vi "Main.vi"() -> ()   [LabVIEW 2021]
doc: "This Continuous Measurement sample project is based on the Queued Message Handler template.\n\nThe Event Handling Loop generates messages based on user interface actions.\n\nThe Message Handling Loop processes messages generated by the Event Handling Loop, or by other messages. There are also Acquisition and Logging message handling loop subVIs, and a chart updating loop."
uses:
  controls/Acquisition Status.ctl
  controls/UI Data.ctl
  controls/Acquired Data.ctl
  controls/UI State.ctl
  support/Message Queue/Enqueue Message (Single).vi
  support/Message Queue/Enqueue Message (Array).vi
  <vilib>/Utility/error.llb/Error Cluster From Error Code.vi
  <vilib>/ErrorRing/Error Ring.xnode
  Acquisition/Acquisition.lvlib
  Logging/Logging.lvlib
  Settings/Settings.lvlib
  support/User Event - Stop/User Event - Stop.lvlib
  support/Message Queue/Message Queue.lvlib
  Settings/Settings Dialog.vi
  Diagnostics/Diagnostics.lvlib
panel:
  out "Data":waveform(dbl)[](graph)
  in  "Save Now":bool
  in  "Settings":bool
  in  "Start":bool
  in  "Stop":bool
  out "Acquisition status":T1
  out "Status":string
  in  "Exit":bool
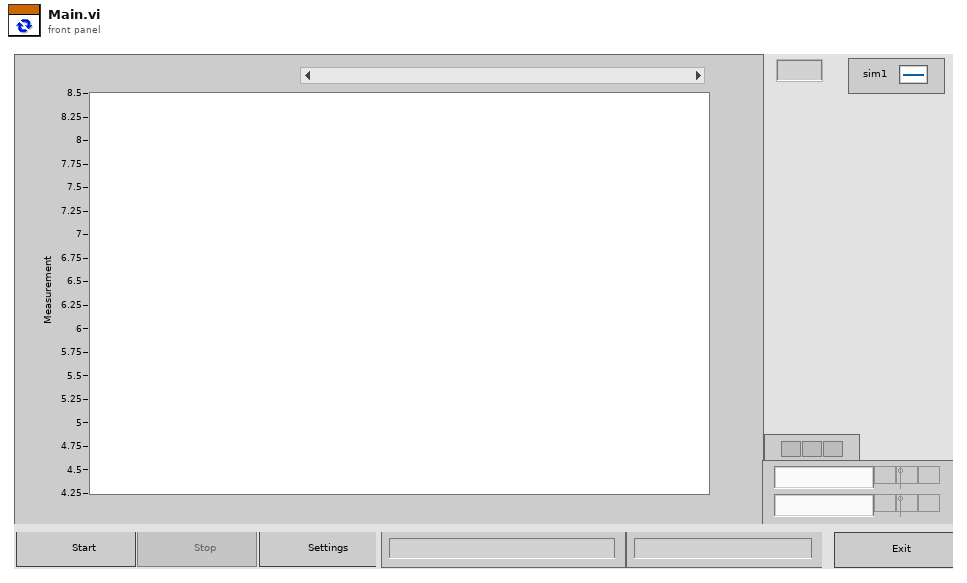
[diagram p1: front panel]
types:
  T1 = typedef "Acquisition Status.ctl" = string
  T2 = typedef "UI State.ctl" = enum16{"Idle", "Acquiring and Logging", "Waiting for Exit", "Waiting for Exit (Acq Stopped)", "Waiting for Exit (Log Stopped)", "Waiting for Stop", "Waiting for Stop (Acq Stopped)", "Waiting for Stop (Log Stopped)"}
  T3 = typedef "Acquired Data.ctl" = cluster{"Waveform Array":waveform(dbl)[]}
  T4 = typedef "UI Data.ctl" = cluster{"Start Ref":refnum<vi>, "Stop Ref":refnum<vi>, "Settings Ref":refnum<vi>, "Exit Ref":refnum<vi>, "Status Ref":refnum<vi>, "Data Ref":refnum<vi>, "Save Ref":refnum<vi>}
  T5 = typedef "Message Queue.lvlib/All Message Queues.ctl" = cluster{"UI":refnum<queue>, "Acquisition":refnum<queue>, "Logging":refnum<queue>, "Diagnostic":refnum<queue>}
  T6 = typedef "Settings.lvlib/Settings.ctl" = cluster{"IO":T7, "Log":T13, "Debug":T14}
  T7 = typedef "Acquisition.lvlib/Hardware Configuration.ctl" = cluster{"Channel Settings":T8[], "Sensor Intervals":T10[], "Sensor Token":T12}
  T8 = typedef "Acquisition.lvlib/Channel Settings.ctl" = cluster{"Name":string, "Terminal Information":cluster{"IO Device":T9, "Channel Number":i32}, "Calibration Information":cluster{"Excitation Voltage":dbl, "Calibration Factor":dbl, "Zero Value":dbl, "Calibration Formula":string}}
  T9 = typedef "Acquisition.lvlib/IO Device.ctl" = enum16{"none", "9219", "9401"}
  T10 = typedef "Interval Timer.lvlib/Repeat Interval.ctl" = cluster{"Interval":T11, "Count":i32}
  T11 = typedef "Interval Timer.lvlib/Interval Length.ctl" = enum16{"Manual control", "1 second", "10 seconds", "30 seconds", "60 seconds", "600 seconds", "1200 seconds", "3600 seconds"}
  T12 = typedef "Interval Timer.lvlib/Interval Token.ctl" = cluster{"Next reading in ms":u32, "Interval Index":i32, "Interval Occurrence":i32}
  T13 = typedef "Logging.lvlib/Logging Configuration.ctl" = cluster{"Path":path, "Spreadsheet":refnum<file>, "Append":bool}
  T14 = typedef "Diagnostics.lvlib/Diagnostics Configuration.ctl" = cluster{"Messages":refnum<file>}
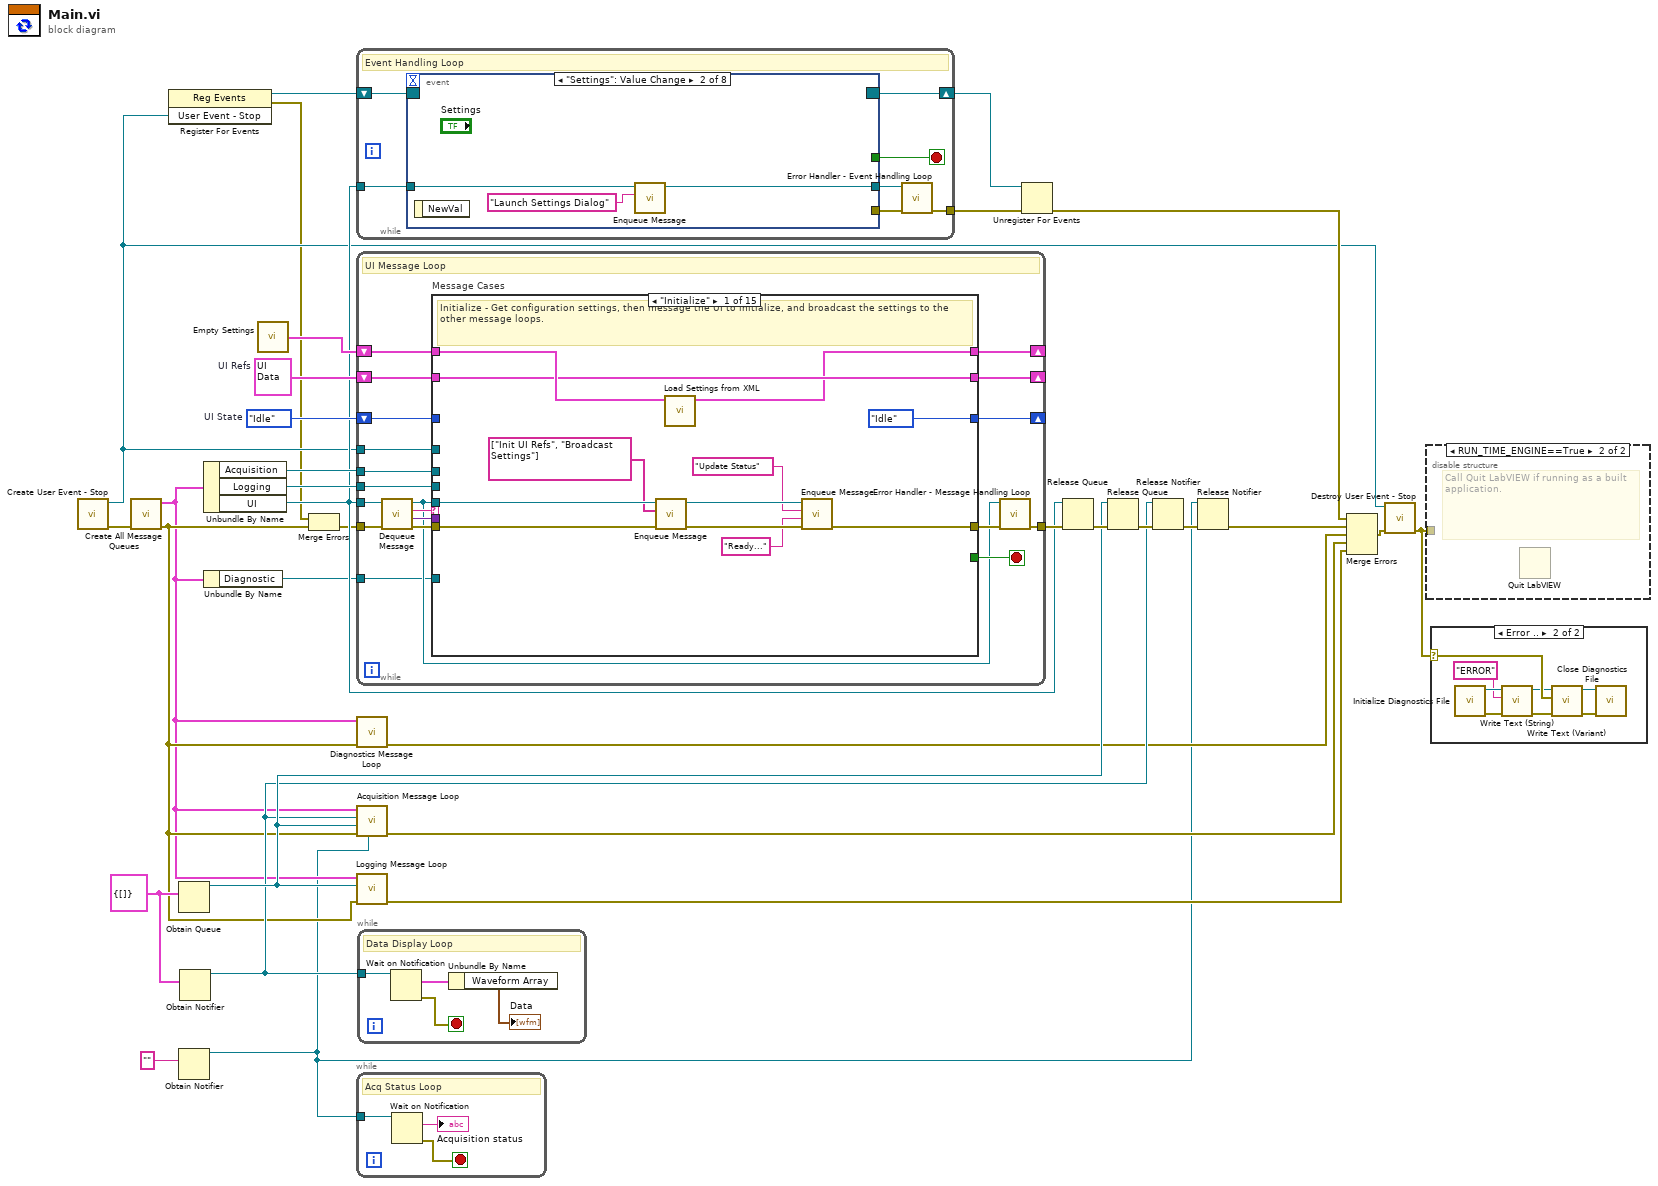
[diagram p0: block diagram]
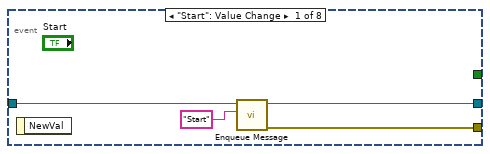
[diagram p4: hidden frame]
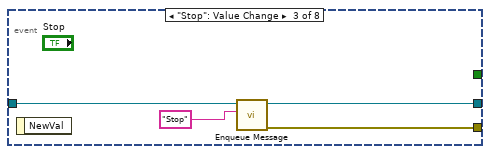
[diagram p5: hidden frame]
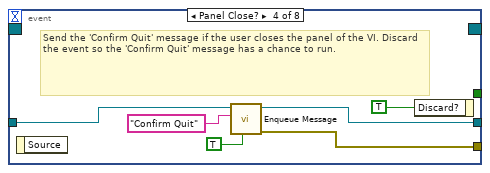
[diagram p6: hidden frame]
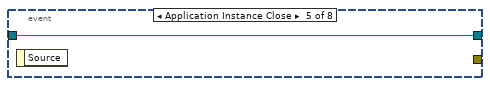
[diagram p7: hidden frame]
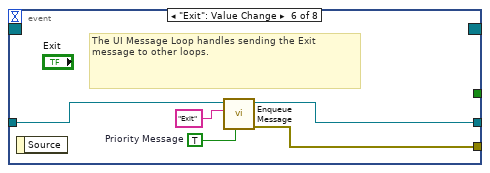
[diagram p8: hidden frame]
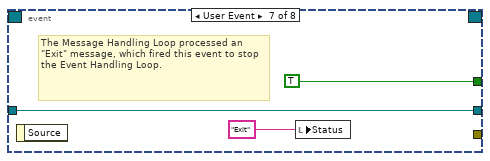
[diagram p9: hidden frame]
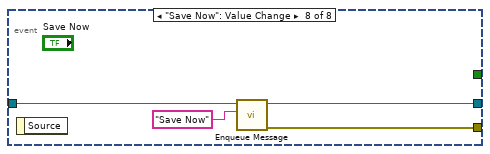
[diagram p10: hidden frame]
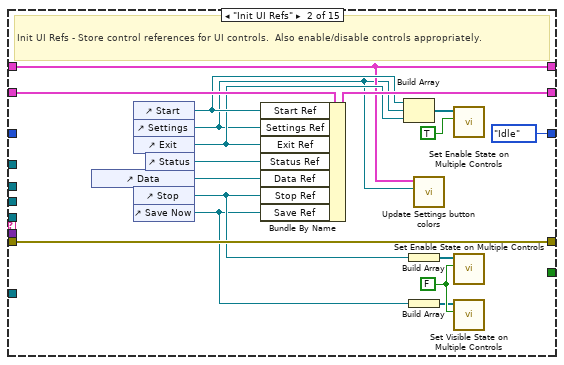
[diagram p11: hidden frame]
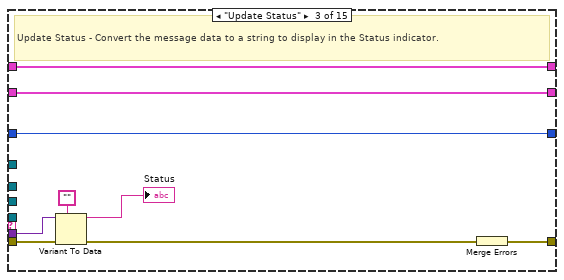
[diagram p12: hidden frame]
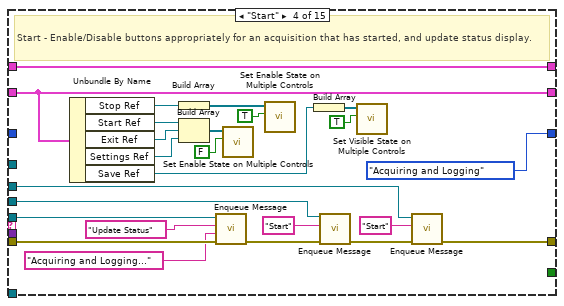
[diagram p13: hidden frame]
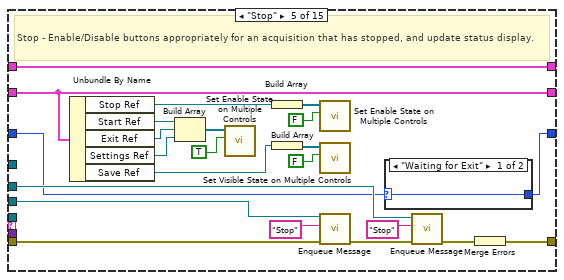
[diagram p14: hidden frame]
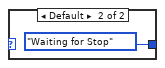
[diagram p15: hidden frame]
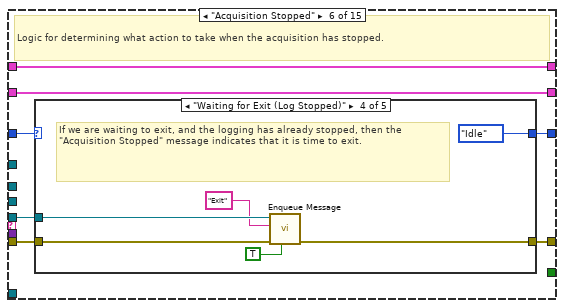
[diagram p16: hidden frame]
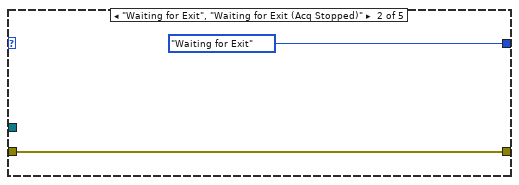
[diagram p18: hidden frame]
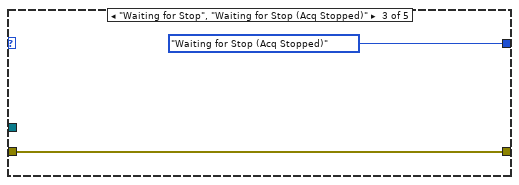
[diagram p19: hidden frame]
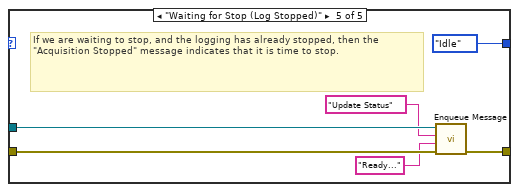
[diagram p20: hidden frame]
diagram:
  w21 = UI_State."Idle"  # UI State
  w14 = T3 {"Waveform Array"=[]}
  w24 = T4 {"Start Ref"=refnum, "Stop Ref"=refnum, "Settings Ref"=refnum, "Exit Ref"=refnum, "Status Ref"=refnum, "Data Ref"=refnum, "Save Ref"=refnum}  # UI Refs
  n1 = call "Create User Event - Stop.vi"() -> ("error out"=w29:errorcluster, "User Event - Stop"=w12:refnum<user-event>)  [unwired: 10 in]
  n2 = call "Create All Message Queues.vi"("error in (no error)"=w29) -> ("error out"=w8:errorcluster, "Message Queues out"=w7:T5)  [unwired: 9 in]
  n3 = register-events(w12) -> (reference out=w13:refnum<event-registration>, error out=w10:errorcluster)  [unwired: 2 in]
  n4 = Obtain Queue(element data type=w14) -> (queue out=w16:refnum<queue>)  [unwired: 4 in, 2 out]
  n5 = Obtain Notifier(notification data type=T1 "") -> (notifier out=w1:refnum<notifier>)  [unwired: 3 in, 2 out]
  n6 = Obtain Notifier(notification data type=w14) -> (notifier out=w15:refnum<notifier>)  [unwired: 3 in, 2 out]
  n7 = Unbundle By Name(w7) -> ("Acquisition"=w23:refnum<queue>, "Logging"=w22:refnum<queue>, "UI"=w19:refnum<queue>)
  n8 = Unbundle By Name(w7) -> ("Diagnostic"=w9:refnum<queue>)
  n9 = call "Empty Settings.vi"() -> ("Settings"=w27:T6)
  n10 = Merge Errors(w10, w8) -> (w11:errorcluster)
  n11 = while {
    tunnel: w19 -> [w38]
    tunnel: [w35] -> w31
    shift-right: [w37] -> w25
    shift-left: w13 -> [w39]
    stop <- w36 stop-if-true
    # "Event Handling Loop"
    n12 = event shown="[1] \"Settings\": Value Change" {
      selector: w39 -> [_ _ _ _ _ _ _ _]
      dyn-events: [_ _ _ _ _ _ _ _] -> w37
      timeout: _ -> [_ _ _ _ _ _ _ _]
      tunnel: [_ _ _ _ _ _ TRUE ("Discard?") _] -> w36
      tunnel: w38 -> [w43 w45 w49 w54 w57 w59 w63 w69]
      tunnel: [w41 _ w48 w52 _ w62 _ w67] -> w34
      tunnel: [w40 w44 w47 w53 w57 w58 w63 w68] -> w33
      event "Start": Value Change {
        n13 = event-data() -> ()  [unwired: 1 in, 1 out]
        n14 = call-poly "Enqueue Message.vi"("Message"="Start", "Message Queue"=w43) -> ("error out"=w41:errorcluster, "dup Message Queue"=w40:refnum<queue>)  [unwired: 8 in]
      }
      event "Settings": Value Change {
        n15 = event-data() -> ()  [unwired: 1 in, 1 out]
        n16 = call-poly "Enqueue Message.vi"("Message"="Launch Settings Dialog", "Message Queue"=w45) -> ("dup Message Queue"=w44:refnum<queue>)  [unwired: 8 in, 1 out]
      }
      event "Stop": Value Change {
        n17 = event-data() -> ()  [unwired: 1 in, 1 out]
        n18 = call-poly "Enqueue Message.vi"("Message"="Stop", "Message Queue"=w49) -> ("error out"=w48:errorcluster, "dup Message Queue"=w47:refnum<queue>)  [unwired: 8 in]
      }
      event Panel Close? {
        # "Send the 'Confirm Quit' message if the user closes the panel of the VI. Discard the event so the 'Confirm Quit' message has a chance to run."
        n19 = event-data() -> ()  [unwired: 1 in, 1 out]
        n20 = call-poly "Enqueue Message.vi"("Priority Message? (F)"=TRUE, "Message"="Confirm Quit", "Message Queue"=w54) -> ("error out"=w52:errorcluster, "dup Message Queue"=w53:refnum<queue>)  [unwired: 7 in]
        n21 = event-data("Discard?"=TRUE) -> ()  [unwired: 1 in, 1 out]
      }
      event Application Instance Close {
        n22 = event-data() -> ()  [unwired: 1 in, 1 out]
      }
      event "Exit": Value Change {
        w60 = TRUE  # Priority Message
        # "The UI Message Loop handles sending the Exit message to other loops."
        n23 = event-data() -> ()  [unwired: 1 in, 1 out]
        n24 = call-poly "Enqueue Message.vi"("Priority Message? (F)"=w60, "Message"="Exit", "Message Queue"=w59) -> ("error out"=w62:errorcluster, "dup Message Queue"=w58:refnum<queue>)  [unwired: 7 in]
      }
      event User Event {
        # "The Message Handling Loop processed an \"Exit\" message, which fired this event to stop the Event Handling Loop."
        n25 = event-data() -> ()  [unwired: 1 in, 1 out]
        n26 = local write "Status"("Exit" ("Exit String")) -> ()
      }
      event "Save Now": Value Change {
        n27 = event-data() -> ()  [unwired: 1 in, 1 out]
        n28 = call-poly "Enqueue Message.vi"("Message"="Save Now", "Message Queue"=w69) -> ("error out"=w67:errorcluster, "dup Message Queue"=w68:refnum<queue>)  [unwired: 8 in]
      }
    }
    n29 = call "Error Handler - Event Handling Loop.vi"("error in (no error)"=w34, "Message Queue"=w33) -> ("dup error in"=w35:errorcluster)  [unwired: 8 in, 1 out]
  }
  n30 = while {
    tunnel: w19 -> [w82]
    tunnel: w12 -> [w87]
    shift-right: [w81] -> _
    shift-left: w27 -> [w80]
    shift-right: [w78] -> _
    shift-left: w24 -> [w79]
    tunnel: w23 -> [w77]
    tunnel: w22 -> [w76]
    shift-right: [w71] -> _
    shift-left: w21 -> [w72]
    tunnel: w11 -> [w86]
    tunnel: [w75] -> w32
    tunnel: w9 -> [w70]
    stop <- w88 stop-if-true
    # "UI Message Loop"
    n31 = call "Dequeue Message.vi"("error in (no error)"=w86, "Message Queue"=w82) -> ("error out"=w85:errorcluster, "Message Data"=w83:variant, "Message"=w84:string, "dup Message Queue"=w73:refnum<queue>)  [unwired: 6 in]
    n32 = case "Message Cases" shown="\"Initialize\"" w84 {
      selector: w84 -> [_ _ _ _ _ _ _ _ _ _ _ _ _ _ w330]
      tunnel: w73 -> [w93 _ _ w151 _ w179 w204 _ w248 _ w269 _ _ _ _]
      tunnel: w85 -> [w92 w117 w125 w150 w173 w180 w205 w239 w250 w257 w268 w307 w320 w323 _]
      tunnel: [w97 w117 w126 w133 w174 w177 w202 w231 w243 w260 w267 w314 w319 w328 w329] -> w74
      tunnel: [_ _ _ _ _ _ _ _ _ _ _ TRUE _ _ _] -> w88
      tunnel: w83 -> [_ _ w124 _ _ _ _ _ _ w261 _ w305 _ _ _]
      tunnel: w87 -> [_ _ _ _ _ _ _ _ _ _ _ w296 _ _ _]
      tunnel: [w89 w102 w120 w149 w172 w183 w208 w227 w247 w265 w272 w300 w318 w327 w333] -> w81
      tunnel: w80 -> [w100 w102 w120 w149 w172 w183 w208 w227 w251 w265 w272 w300 w318 w327 w333]
      tunnel: w79 -> [w94 w116 w119 w146 w171 w182 w207 w230 w245 w264 w271 w295 w317 w326 w332]
      tunnel: [w94 w113 w119 w146 w171 w182 w207 w230 w245 w264 w271 w295 w317 w326 w332] -> w78
      tunnel: w77 -> [_ _ _ w132 w158 _ _ w238 _ _ _ w313 _ w321 _]
      tunnel: w76 -> [_ _ _ w135 w161 _ _ w237 _ _ _ w312 _ _ _]
      tunnel: w72 -> [_ _ w118 _ w155 w181 w206 w236 w244 w259 w270 _ w316 w325 w331]
      tunnel: [UI_State."Idle" ("UI State") UI_State."Idle" ("UI State") w118 UI_State."Acquiring and Logging" ("UI State") w156 w178 w203 w236 w244 w259 w266 UI_State."Idle" ("UI State") w316 w325 w331] -> w71
      tunnel: w70 -> [_ _ _ _ _ _ _ w235 _ _ _ w303 _ _ _]
      frame "Initialize" {
        # "Initialize - Get configuration settings, then message the UI to initialize, and broadcast the settings to the other message loops."
        n33 = call-poly "Enqueue Message.vi"("error in (no error)"=w92, "Message Array"=string[] ["Init UI Refs", "Broadcast Settings"], "Message Queue"=w93) -> ("error out"=w99:errorcluster, "dup Message Queue"=w98:refnum<queue>)  [unwired: 7 in]
        n34 = call "Load Settings from XML.vi"("Settings in"=w100) -> ("Settings out"=w89:T6)  [unwired: 9 in, 1 out]
        n35 = call-poly "Enqueue Message.vi"("error in (no error)"=w99, "Message Data"="Ready..." ("Ready..."), "Message"="Update Status", "Message Queue"=w98) -> ("error out"=w97:errorcluster)  [unwired: 6 in, 1 out]
      }
      frame "Init UI Refs" {
        w105 = FALSE ("Enable?")
        # "Init UI Refs - Store control references for UI controls.  Also enable/disable controls appropriately."
        n36 = control-ref of="Data"() -> (w114:refnum<vi>)
        n37 = control-ref of="Start"() -> (w109:refnum<vi>)
        n38 = control-ref of="Settings"() -> (w101:refnum<vi>)
        n39 = control-ref of="Exit"() -> (w108:refnum<vi>)
        n40 = control-ref of="Stop"() -> (w106:refnum<vi>)
        n41 = control-ref of="Save Now"() -> (w103:refnum<vi>)
        n42 = control-ref of="Status"() -> (w115:refnum<vi>)
        n43 = Bundle By Name(cluster=w116, "Start Ref"=w109, "Settings Ref"=w101, "Exit Ref"=w108, "Status Ref"=w115, "Data Ref"=w114, "Stop Ref"=w106, "Save Ref"=w103) -> (w113:T4)
        n44 = Build Array(w109, w101, w108) -> (w111:refnum<vi>[])
        n45 = Build Array(w106) -> (w110:refnum<vi>[])
        n46 = Build Array(w103) -> (w104:refnum<vi>[])
        n47 = call "Update Settings button colors.vi"("Bool Refnum"=w101, "Settings in"=w102) -> ()  [unwired: 8 in, 2 out]
        n48 = call "Set Enable State on Multiple Controls.vi"("Enable?"=TRUE, "Controls"=w111) -> ()  [unwired: 9 in, 1 out]
        n49 = call "Set Enable State on Multiple Controls.vi"("Enable?"=w105, "Controls"=w110) -> ()  [unwired: 9 in, 1 out]
        n50 = call "Set Visible State on Multiple Controls.vi"("Visible?"=w105, "Controls"=w104) -> ()  [unwired: 10 in]
      }
      frame "Update Status" {
        # "Update Status - Convert the message data to a string to display in the Status indicator."
        n51 = Variant To Data(error in=w125, type="", Variant=w124) -> (data=→"Status":string, error out=w122:errorcluster)
        n52 = Merge Errors(w122) -> (w126:errorcluster)
      }
      frame "Start" {
        # "Start - Enable/Disable buttons appropriately for an acquisition that has started, and update status display."
        n53 = Unbundle By Name(w146) -> ("Stop Ref"=w141:refnum<vi>, "Start Ref"=w140:refnum<vi>, "Exit Ref"=w139:refnum<vi>, "Settings Ref"=w138:refnum<vi>, "Save Ref"=w128:refnum<vi>)
        n54 = Build Array(w141) -> (w143:refnum<vi>[])
        n55 = Build Array(w140, w139, w138) -> (w144:refnum<vi>[])
        n56 = call-poly "Enqueue Message.vi"("error in (no error)"=w150, "Message Data"="Acquiring and Logging..." ("Acquiring and Logging..."), "Message"="Update Status", "Message Queue"=w151) -> ("error out"=w137:errorcluster)  [unwired: 6 in, 1 out]
        n57 = call "Set Enable State on Multiple Controls.vi"("Enable?"=FALSE, "Controls"=w144) -> ()  [unwired: 9 in, 1 out]
        n58 = call "Set Enable State on Multiple Controls.vi"("Enable?"=TRUE, "Controls"=w143) -> ()  [unwired: 9 in, 1 out]
        n59 = Build Array(w128) -> (w129:refnum<vi>[])
        n60 = call-poly "Enqueue Message.vi"("error in (no error)"=w137, "Message"="Start", "Message Queue"=w135) -> ("error out"=w134:errorcluster)  [unwired: 7 in, 1 out]
        n61 = call "Set Visible State on Multiple Controls.vi"("Visible?"=TRUE ("Visble?"), "Controls"=w129) -> ()  [unwired: 10 in]
        n62 = call-poly "Enqueue Message.vi"("error in (no error)"=w134, "Message"="Start", "Message Queue"=w132) -> ("error out"=w133:errorcluster)  [unwired: 7 in, 1 out]
      }
      frame "Stop" {
        # "Stop - Enable/Disable buttons appropriately for an acquisition that has stopped, and update status display."
        n63 = Unbundle By Name(w171) -> ("Stop Ref"=w166:refnum<vi>, "Start Ref"=w165:refnum<vi>, "Exit Ref"=w164:refnum<vi>, "Settings Ref"=w163:refnum<vi>, "Save Ref"=w152:refnum<vi>)
        n64 = Build Array(w165, w164, w163) -> (w169:refnum<vi>[])
        n65 = call "Set Enable State on Multiple Controls.vi"("Enable?"=TRUE, "Controls"=w169) -> ()  [unwired: 9 in, 1 out]
        n66 = Build Array(w166) -> (w168:refnum<vi>[])
        n67 = Build Array(w152) -> (w154:refnum<vi>[])
        n68 = call "Set Enable State on Multiple Controls.vi"("Enable?"=FALSE, "Controls"=w168) -> ()  [unwired: 9 in, 1 out]
        n69 = call "Set Visible State on Multiple Controls.vi"("Visible?"=FALSE ("Enable?"), "Controls"=w154) -> ()  [unwired: 10 in]
        n70 = call-poly "Enqueue Message.vi"("error in (no error)"=w173, "Message"="Stop", "Message Queue"=w161) -> ("error out"=w160:errorcluster)  [unwired: 7 in, 1 out]
        n71 = case shown="\"Waiting for Exit\"" w155 {
          selector: w155 -> [w175 _]
          tunnel: [w175 UI_State."Waiting for Stop" ("UI State")] -> w156
          frame "Waiting for Exit" {
          }
          frame Default {
          }
        }
        n72 = call-poly "Enqueue Message.vi"("error in (no error)"=w160, "Message"="Stop", "Message Queue"=w158) -> ("error out"=w159:errorcluster)  [unwired: 7 in, 1 out]
        n73 = Merge Errors(w159) -> (w174:errorcluster)
      }
      frame "Acquisition Stopped" {
        # "Logic for determining what action to take when the acquisition has stopped."
        n74 = case shown="\"Waiting for Exit (Log Stopped)\"" w181 {
          selector: w181 -> [w185 _ _ _ _]
          tunnel: w180 -> [w184 w187 w189 w195 w201]
          tunnel: w179 -> [_ _ _ w193 w198]
          tunnel: [w185 UI_State."Waiting for Exit" ("UI State") UI_State."Waiting for Stop (Acq Stopped)" ("UI State") UI_State."Idle" ("UI State") UI_State."Idle" ("UI State")] -> w178
          tunnel: [w184 w187 w189 w194 w199] -> w177
          frame Default {
          }
          frame "Waiting for Exit", "Waiting for Exit (Acq Stopped)" {
          }
          frame "Waiting for Stop", "Waiting for Stop (Acq Stopped)" {
          }
          frame "Waiting for Exit (Log Stopped)" {
            # "If we are waiting to exit, and the logging has already stopped, then the \"Acquisition Stopped\" message indicates that it is time to exit."
            n75 = call-poly "Enqueue Message.vi"("Priority Message? (F)"=TRUE, "error in (no error)"=w195, "Message"="Exit", "Message Queue"=w193) -> ("error out"=w194:errorcluster)  [unwired: 6 in, 1 out]
          }
          frame "Waiting for Stop (Log Stopped)" {
            # "If we are waiting to stop, and the logging has already stopped, then the \"Acquisition Stopped\" message indicates that it is time to stop."
            n76 = call-poly "Enqueue Message.vi"("error in (no error)"=w201, "Message Data"="Ready..." ("Ready..."), "Message"="Update Status", "Message Queue"=w198) -> ("error out"=w199:errorcluster)  [unwired: 6 in, 1 out]
          }
        }
      }
      frame "Logging Stopped" {
        # "Logic for determining what action to take when the logging has stopped."
        n77 = case shown="\"Waiting for Exit (Acq Stopped)\"" w206 {
          selector: w206 -> [w210 _ _ _ _]
          tunnel: w205 -> [w209 w212 w214 w220 w223]
          tunnel: w204 -> [_ _ _ w218 w222]
          tunnel: [w210 UI_State."Waiting for Exit (Log Stopped)" ("UI State") UI_State."Waiting for Stop (Log Stopped)" ("UI State") UI_State."Idle" ("UI State") UI_State."Idle" ("UI State")] -> w203
          tunnel: [w209 w212 w214 w219 w221] -> w202
          frame Default {
          }
          frame "Waiting for Exit", "Waiting for Exit (Log Stopped)" {
          }
          frame "Waiting for Stop", "Waiting for Stop (Log Stopped)" {
          }
          frame "Waiting for Exit (Acq Stopped)" {
            # "If we are waiting to exit, and the acquisition has already stopped, then the \"Logging Stopped\" message indicates that it is time to exit."
            n78 = call-poly "Enqueue Message.vi"("Priority Message? (F)"=TRUE, "error in (no error)"=w220, "Message"="Exit", "Message Queue"=w218) -> ("error out"=w219:errorcluster)  [unwired: 6 in, 1 out]
          }
          frame "Waiting for Stop (Acq Stopped)" {
            # "If we are waiting to stop, and the acquisition has already stopped, then the \"Logging Stopped\" message indicates that it is time to stop."
            n79 = call-poly "Enqueue Message.vi"("error in (no error)"=w223, "Message Data"="Ready..." ("Ready..."), "Message"="Update Status", "Message Queue"=w222) -> ("error out"=w221:errorcluster)  [unwired: 6 in, 1 out]
          }
        }
      }
      frame "Broadcast settings" {
        w234 = "Update Settings" ("Message")
        # "Broadcast settings - Send the 'Update Settings' message to the Logging and Acquisition message loops."
        n80 = Unbundle By Name(w227) -> ("IO"=w241:T7)
        n81 = call-poly "Enqueue Message.vi"("Message Data"=w241, "Message"=w234, "Message Queue"=w238) -> ("error out"=w242:errorcluster)  [unwired: 7 in, 1 out]
        n82 = call-poly "Enqueue Message.vi"("Message Data"=w227, "Message"=w234, "Message Queue"=w235) -> ("error out"=w233:errorcluster)  [unwired: 7 in, 1 out]
        n83 = call-poly "Enqueue Message.vi"("error in (no error)"=w242, "Message Data"=w227, "Message"=w234, "Message Queue"=w237) -> ("error out"=w240:errorcluster)  [unwired: 6 in, 1 out]
        n84 = control-ref of="Data"() -> (w228:refnum<vi>)
        n85 = Merge Errors(w240, w239, w233) -> (w232:errorcluster)
        n86 = Unbundle By Name(w230) -> ("Settings Ref"=w229:refnum<vi>)
        n87 = call "Set Plot Count.vi"("Settings"=w227, "Waveform Chart ref"=w228) -> ()  [unwired: 10 in]
        n88 = call "Update Settings button colors.vi"("error in (no error)"=w232, "Bool Refnum"=w229, "Settings in"=w227) -> ("error out"=w231:errorcluster)  [unwired: 7 in, 1 out]
      }
      frame "Launch Settings Dialog" {
        # "Launch Settings Dialog - Launch the Settings Dialog when the user clicks the 'Settings' button."
        n89 = call-by-ref "?"("error in (no error)"=w250, "Settings in"=w251) -> ("error out"=w246:errorcluster, "Cancelled?"=w249:bool, "Settings out"=w247:T6)  [unwired: 8 in, 3 out]
        n90 = case shown="False" w249 {
          tunnel: w248 -> [w255 _]
          tunnel: w246 -> [w254 w256]
          tunnel: [w253 w256] -> w243
          frame False {
            n91 = call-poly "Enqueue Message.vi"("error in (no error)"=w254, "Message"="Broadcast Settings", "Message Queue"=w255) -> ("error out"=w253:errorcluster)  [unwired: 7 in, 1 out]
          }
          frame True {
          }
        }
      }
      frame "Error" {
        # "Error - Display an error dialog. This message is sent by the \"Error Handler\" VIs at the end of other loops in this application."
        n92 = Variant To Data(error in=w257, type=errorcluster {"status"=FALSE, "code"=0, "source"=""} ("error constant"), Variant=w261) -> (data=w258:errorcluster, error out=w262:errorcluster)
        n93 = call <vilib>:"Simple Error Handler.vi"("error in (no error)"=w258) -> ()  [unwired: 4 in, 5 out]
        n94 = Merge Errors(w262) -> (w260:errorcluster)
      }
      frame "Confirm Quit" {
        # "Confirm Quit - Message that can confirm whether or not the user wants to exit the application."
        n95 = case shown="\"Acquiring and Logging\"" w270 {
          tunnel: w269 -> [w278 w282]
          tunnel: w268 -> [w277 w281]
          tunnel: [w276 w280] -> w267
          tunnel: [UI_State."Idle" ("UI State") w279] -> w266
          frame Default {
            # "If 'Confirm Quit' comes in while the system is idle, there is no need for a confirmation message."
            n96 = call-poly "Enqueue Message.vi"("Priority Message? (F)"=TRUE, "error in (no error)"=w277, "Message"="Exit", "Message Queue"=w278) -> ("error out"=w276:errorcluster)  [unwired: 6 in, 1 out]
          }
          frame "Acquiring and Logging" {
            n97 = Two Button Dialog(message="Are you sure you want to quit while the acquisition is running?" ("Confirm Quit Message"), 1:"No" ("No"), 2:"Yes" ("Yes")) -> (T button?=w283:bool)
            n98 = case shown="True" w283 {
              tunnel: w282 -> [_ w292]
              tunnel: w281 -> [w288 w293]
              tunnel: [w288 w291] -> w280
              tunnel: [UI_State."Acquiring and Logging" ("UI State") UI_State."Waiting for Exit" ("UI State")] -> w279
              frame False {
                # "User did not want to quit."
              }
              frame True {
                n99 = call-poly "Enqueue Message.vi"("error in (no error)"=w293, "Message"="Stop", "Message Queue"=w292) -> ("error out"=w291:errorcluster)  [unwired: 7 in, 1 out]
              }
            }
          }
        }
      }
      frame "Exit" {
        w299 = TRUE  # Force Default Colors
        w309 = TRUE ("Priority Message? (F)")
        w302 = "Exit" ("Message")
        # "Popup an error dialog if 'Exit' was called as a result of an error."
        # "Stop the VI"
        # "Exit - Send Exit messages to the Acquisition and Logging loops, and fire the user event to stop the Event Handling Loop."
        n100 = Variant To Data(type=errorcluster {"status"=FALSE, "code"=0, "source"=""} ("error constant"), Variant=w305) -> (data=w304:errorcluster)  [unwired: 1 in, 1 out]
        n101 = call <vilib>:"Simple Error Handler.vi"("error in (no error)"=w304) -> ()  [unwired: 4 in, 5 out]
        n102 = call-poly "Enqueue Message.vi"("Priority Message? (F)"=w309, "error in (no error)"=w307, "Message"=w302, "Message Queue"=w313) -> ("error out"=w310:errorcluster)  [unwired: 6 in, 1 out]
        n103 = call-poly "Enqueue Message.vi"("Message"=w302, "Message Queue"=w303) -> ("error out"=w301:errorcluster)  [unwired: 8 in, 1 out]
        n104 = call-poly "Enqueue Message.vi"("Priority Message? (F)"=w309, "error in (no error)"=w310, "Message"=w302, "Message Queue"=w312) -> ("error out"=w308:errorcluster)  [unwired: 6 in, 1 out]
        n105 = Unbundle By Name(w295) -> ("Settings Ref"=w294:refnum<vi>)
        n106 = Merge Errors(w308, w301) -> (w298:errorcluster)
        n107 = call "Update Settings button colors.vi"("error in (no error)"=w298, "Force Default Colors (F)"=w299, "Bool Refnum"=w294, "Settings in"=w300) -> ("error out"=w297:errorcluster)  [unwired: 6 in, 1 out]
        n108 = call "Invoke User Event - Stop.vi"("error in (no error)"=w297, "User Event - Stop"=w296) -> ("error out"=w314:errorcluster)  [unwired: 9 in]
      }
      frame "---Copy This Frame---" {
        # "Duplicate this frame when creating new messages.  Change this comment in the duplicated frame to describe this message."
        n109 = Merge Errors(w320) -> (w319:errorcluster)
      }
      frame "Save Now" {
        # "Take a measurement on-demand."
        n110 = call-poly "Enqueue Message.vi"("error in (no error)"=w323, "Message"="Save Now", "Message Queue"=w321) -> ("error out"=w322:errorcluster)  [unwired: 7 in, 1 out]
        n111 = Merge Errors(w322) -> (w328:errorcluster)
      }
      frame Default {
        # "'Default' case only runs if there is a message that isn't defined in any of the other cases.  Output a programming error."
        n112 = xnode "Error Ring"("parameter 0"=w330) -> ("error out"=w329:errorcluster)
      }
    }
    n113 = call "Error Handler - Message Handling Loop.vi"("error in (no error)"=w74, "Message Queue"=w73) -> ("dup error in"=w75:errorcluster)  [unwired: 8 in, 1 out]
  }
  n114 = call "Diagnostics Message Loop.vi"("error in (no error)"=w8, "Message Queues"=w7) -> ("error out"=w6:errorcluster)  [unwired: 9 in]
  n115 = call "Acquisition Message Loop.vi"("Acquisition Status Notifier"=w1, "error in (no error)"=w8, "Data Queue"=w16, "Data Notifier"=w15, "Message Queues"=w7) -> ("error out"=w30:errorcluster)  [unwired: 6 in]
  n116 = call "Logging Message Loop.vi"("error in (no error)"=w8, "Data Queue"=w16, "Message Queues"=w7) -> ("error out"=w28:errorcluster)  [unwired: 8 in]
  n117 = while {
    tunnel: w1 -> [w341]
    stop <- w343 stop-if-true
    # "Acq Status Loop"
    n118 = Wait on Notification(notifier=w341) -> (notification=→"Acquisition status":T1, error out=w343:errorcluster)  [unwired: 3 in, 2 out]
  }
  n119 = while "Data Display Loop" {
    tunnel: w15 -> [w347]
    stop <- w346 stop-if-true
    # "Data Display Loop"
    n120 = Wait on Notification(notifier=w347) -> (notification=w344:T3, error out=w346:errorcluster)  [unwired: 3 in, 2 out]
    n121 = Unbundle By Name(w344) -> ("Waveform Array"=→"Data":waveform(dbl)[])
  }
  n122 = Unregister For Events(event registration refnum=w25, error in=w31) -> (error out=w26:errorcluster)
  n123 = Release Queue(queue=w19, error in (no error)=w32) -> (error out=w18:errorcluster)  [unwired: 1 in, 2 out]
  n124 = Release Queue(queue=w16, error in (no error)=w18) -> (error out=w17:errorcluster)  [unwired: 1 in, 2 out]
  n125 = Release Notifier(notifier=w15, error in (no error)=w17) -> (error out=w3:errorcluster)  [unwired: 1 in, 2 out]
  n126 = Release Notifier(notifier=w1, error in (no error)=w3) -> (error out=w2:errorcluster)  [unwired: 1 in, 2 out]
  n127 = Merge Errors(w26, w2, w6, w30, w28) -> (w20:errorcluster)
  n128 = call "Destroy User Event - Stop.vi"("error in (no error)"=w20, "User Event - Stop"=w12) -> ("error out"=w5:errorcluster)  [unwired: 9 in]
  n129 = disable-structure shown="RUN_TIME_ENGINE==True" {
    disable-tunnel: w5 -> [_ _]
    frame condition #0 (active) {
    }
    frame condition #1 {
      # "Call Quit LabVIEW if running as a built application."
      n130 = Quit LabVIEW() -> ()  [unwired: 1 in]
    }
  }
  n131 = case shown="Error .." w5 {
    selector: w5 -> [_ w353]
    frame No Error {
    }
    frame Error {
      n132 = call "Initialize Diagnostics File.vi"() -> ("error out"=w352:errorcluster, "diagnostics file"=w349:refnum<file>)  [unwired: 10 in]
      n133 = call "Write Text (String).vi"("error in"=w352, "String"="ERROR", "file in"=w349) -> ("error out"=w351:errorcluster, "file out"=w350:refnum<file>)  [unwired: 7 in]
      n134 = call "Write Text (Variant).vi"("error in"=w351, "Anything"=w353, "file in"=w350) -> ("error out"=w355:errorcluster, "file out"=w354:refnum<file>)  [unwired: 7 in]
      n135 = call "Close Diagnostics File.vi"("error in"=w355, "diagnostics file"=w354) -> ()  [unwired: 8 in, 2 out]
    }
  }
